vi "ControlShooter.vi"(1 "right down":T4, 2 "right up":T4, 3 "latch":T1={"DevStatus"={"status"=FALSE, "code"=0, "source"=""}, "Solenoid Module"=enum."Solenoid Module 1", "Forward Solenoid Channel"=enum."Invalid", "Reverse Solenoid Channel"=enum."Invalid"}, 4 "State":T8) -> ()   [LabVIEW 2013]
uses:
  typedefs/subStates.ctl
  <vilib>/Rock Robotics/WPI/Solenoid/WPI_SolenoidValue.ctl
  <vilib>/Rock Robotics/WPI/DigitalInput/WPI_DigitalInputDevRef.ctl
  <vilib>/Rock Robotics/SystemInterfaces/DIO/FPGA_DIOChannel.ctl
  <vilib>/Rock Robotics/SystemInterfaces/Typedef/FPGA_TypedefDigitalModule.ctl
  <vilib>/Rock Robotics/WPI/Solenoid/WPI_SolenoidDevRef.ctl
  <vilib>/Rock Robotics/SystemInterfaces/Typedef/FPGA_TypedefSolenoidModule.ctl
  <vilib>/Rock Robotics/WPI/Solenoid/WPI_SolenoidChannel.ctl
  typedefs/fg_typedef.ctl
  <vilib>/Rock Robotics/WPI/Solenoid/WPI_SolenoidGetEnum.vi
panel:
  out "To Shooter\nSolenoid Loop":T7=enum."Forward"
  # "unused"
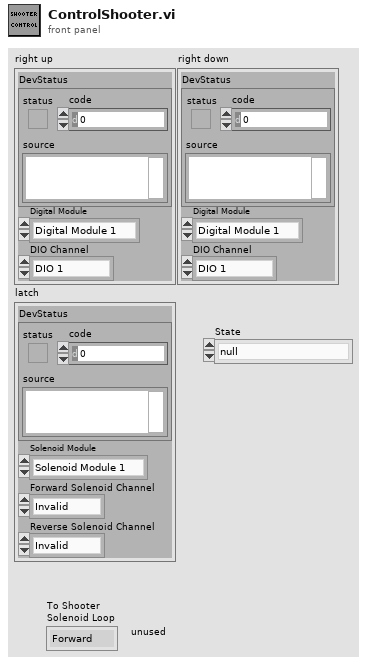
[diagram p1: front panel]
types:
  T1 = typedef "WPI_SolenoidDevRef.ctl" = cluster{"DevStatus":errorcluster, "Solenoid Module":T2, "Forward Solenoid Channel":T3, "Reverse Solenoid Channel":T3}
  T2 = typedef "FPGA_TypedefSolenoidModule.ctl" = enum16{"Solenoid Module 1", "Solenoid Module 2"}
  T3 = typedef "WPI_SolenoidChannel.ctl" = enum8{"Solenoid 1", "Solenoid 2", "Solenoid 3", "Solenoid 4", "Solenoid 5", "Solenoid 6", "Solenoid 7", "Solenoid 8", "Invalid"}
  T4 = typedef "WPI_DigitalInputDevRef.ctl" = cluster{"DevStatus":errorcluster, "DIO Channel":T5, "Digital Module":T6}
  T5 = typedef "FPGA_DIOChannel.ctl" = enum8{"DIO 1", "DIO 2", "DIO 3", "DIO 4", "DIO 5", "DIO 6", "DIO 7", "DIO 8", "DIO 9", "DIO 10", "DIO 11", "DIO 12", "DIO 13", "DIO 14", "Invalid"}
  T6 = typedef "FPGA_TypedefDigitalModule.ctl" = enum16{"Digital Module 1", "Digital Module 2"}
  T7 = typedef "WPI_SolenoidValue.ctl" = enum16{"Off", "On", "Forward", "Reverse"}
  T8 = typedef "subStates.ctl" = enum16{"null", "wait", "driver control", "auto", "manual override", "hold position", "rotate", "pickup", "pass", "load", "goto shoot", "shoot", "cancel", "end"}
  T9 = typedef "fg_typedef.ctl" = enum16{"Get", "Set"}
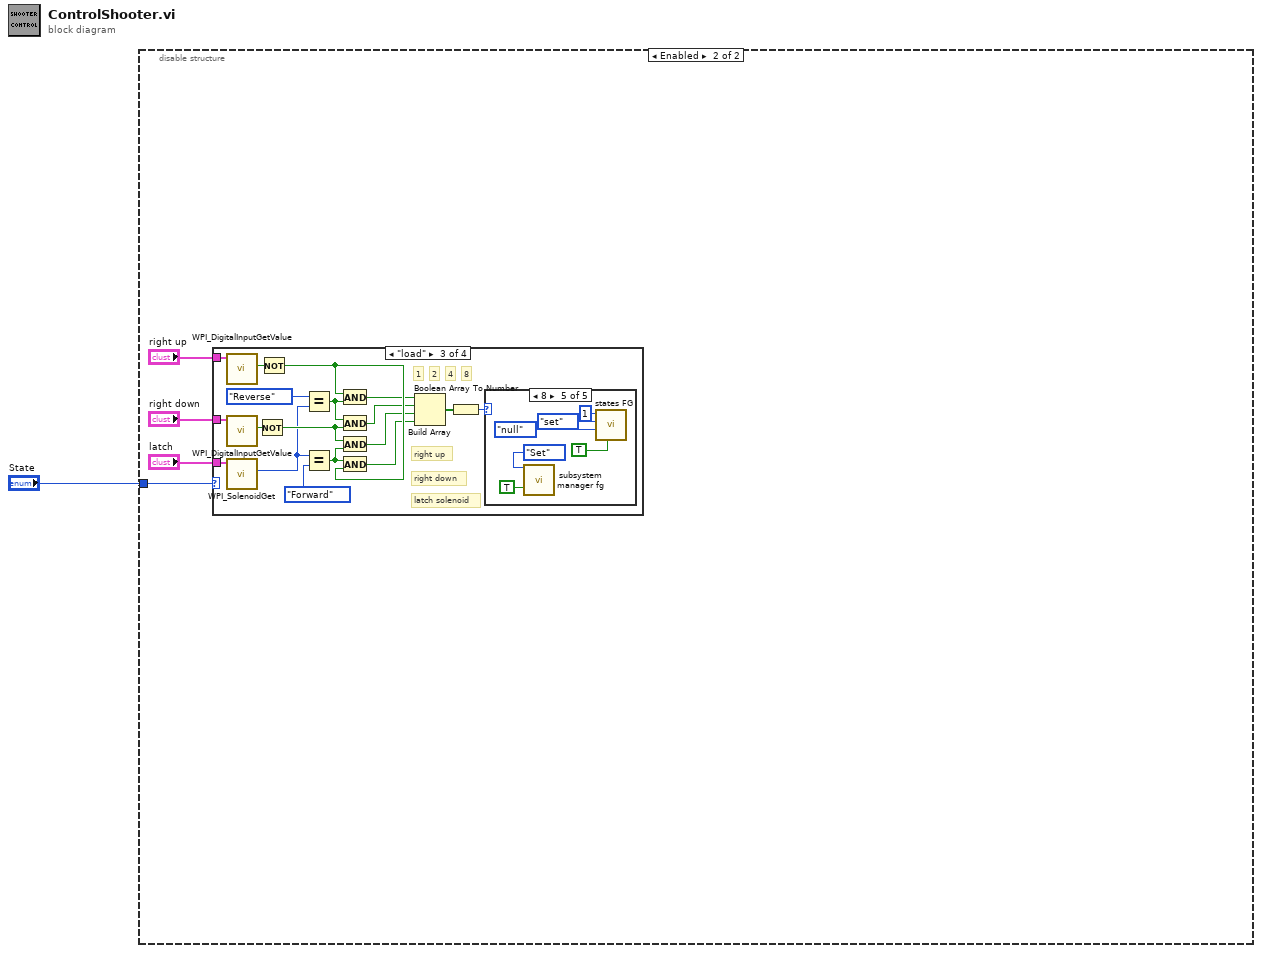
[diagram p0: block diagram]
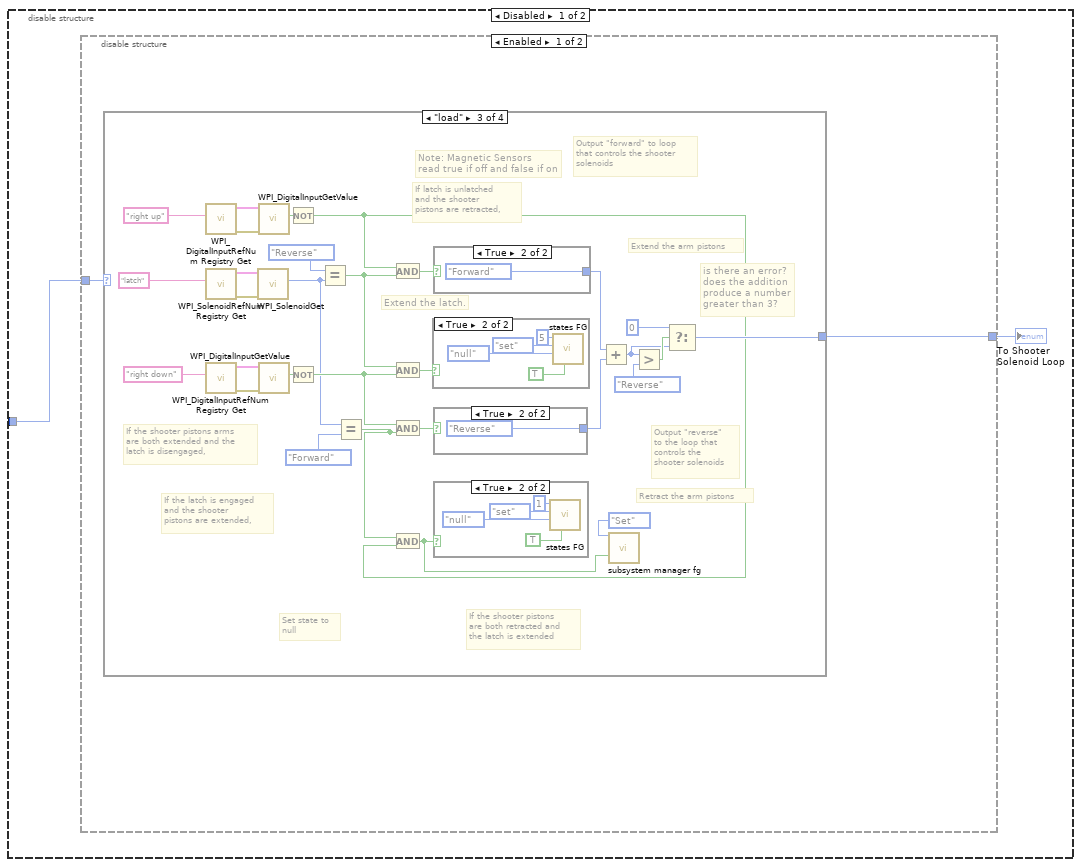
[diagram p2: hidden frame]
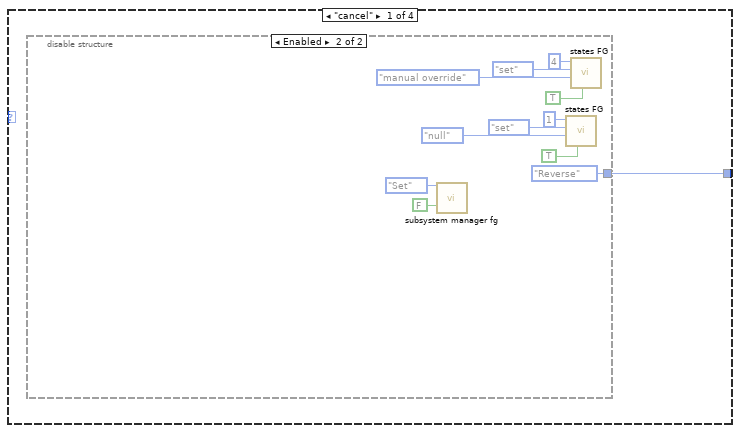
[diagram p3: hidden frame]
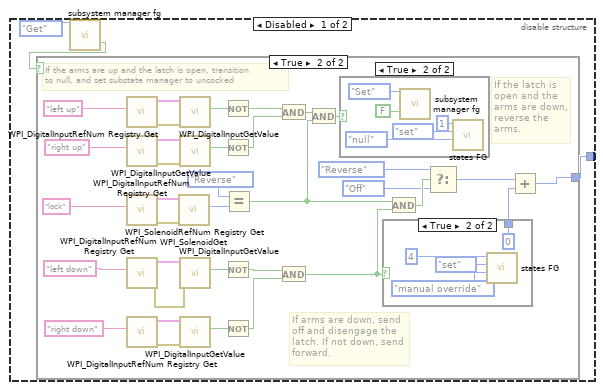
[diagram p4: hidden frame]
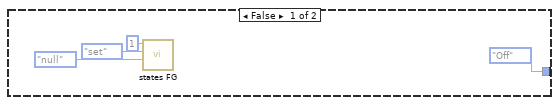
[diagram p5: hidden frame]
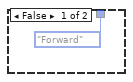
[diagram p7: hidden frame]
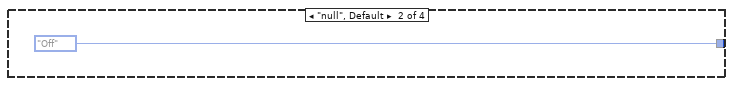
[diagram p8: hidden frame]
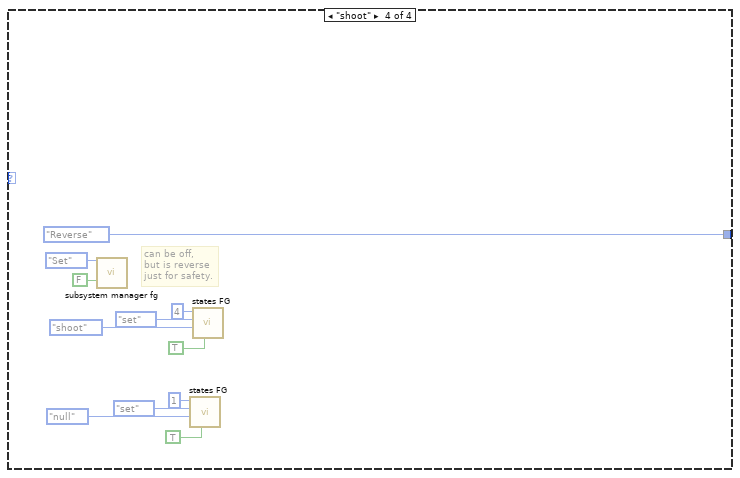
[diagram p13: hidden frame]
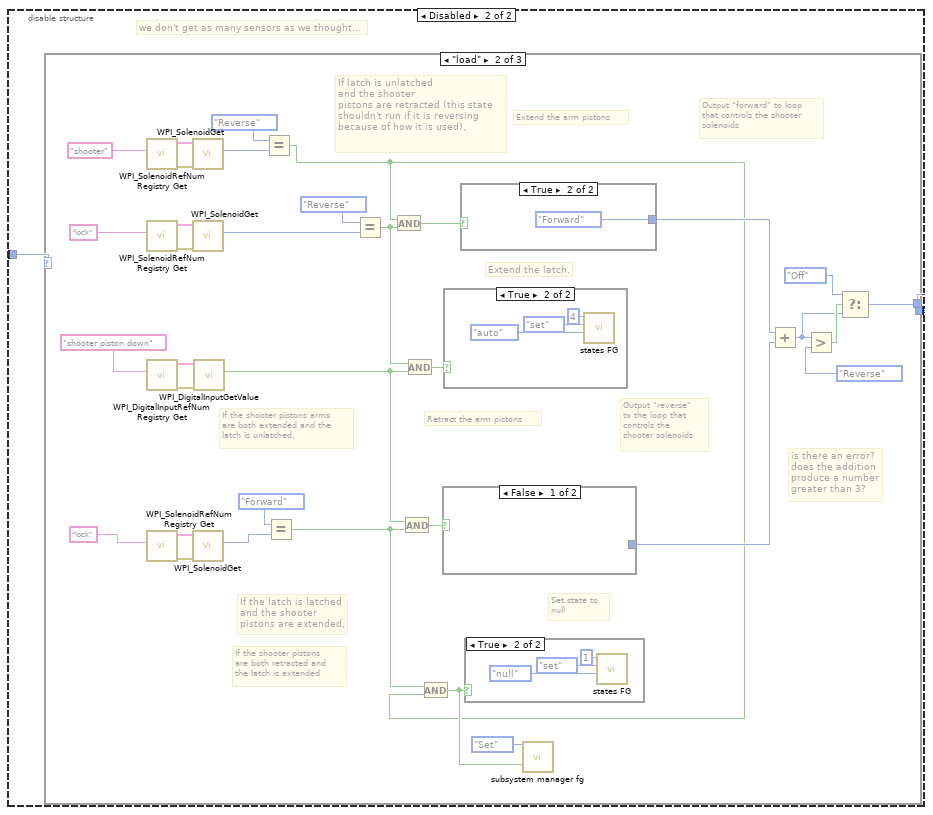
[diagram p14: hidden frame]
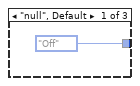
[diagram p15: hidden frame]
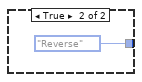
[diagram p17: hidden frame]
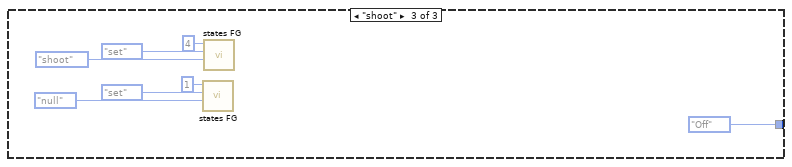
[diagram p20: hidden frame]
diagram:
  n1 = disable-structure shown="Enabled" {
    disable-tunnel: "State" -> [w3 w174]
    frame Disabled {
      n2 = disable-structure shown="Enabled" {
        disable-tunnel: w3 -> [w5 w123]
        disable-tunnel: [w4 w122] -> w2
        frame Enabled {
          n3 = case shown="\"load\"" w5 {
            tunnel: [w6 WPI_SolenoidValue."Off" ("To Shooter\nSolenoid Loop") w81 WPI_SolenoidValue."Reverse" ("To Shooter\nSolenoid Loop")] -> w4
            frame "cancel" {
              n4 = disable-structure shown="Enabled" {
                disable-tunnel: [w7 WPI_SolenoidValue."Reverse" ("To Shooter\nSolenoid Loop")] -> w6
                frame Disabled {
                  n5 = call "subsystem manager fg.vi"("Menu"=fg_typedef."Get") -> ("Shooter Cocked"=w8:bool)  [unwired: 14 in, 4 out]
                  n6 = case shown="True" w8 {
                    tunnel: [WPI_SolenoidValue."Off" ("To Shooter\nSolenoid Loop") w17] -> w7
                    frame False {
                      n7 = call "states FG.vi"("subState in"=subStates."null", "menu (get)"=enum16{"set", "get"}."set", "Loop ID"=1) -> ()  [unwired: 5 in, 4 out]
                    }
                    frame True {
                      # "If the arms are up and the latch is open, transition\nto null, and set substate manager to uncocked"
                      # "If the latch is\nopen and the\narms are down,\nreverse the\narms."
                      # "If arms are down, send\noff and disengage the\nlatch. If not down, send\nforward."
                      n8 = call <vilib>:"WPI_DigitalInputRefNum Registry Get.vi"("refnum name"="left up") -> ("error out"=w35:errorcluster, "DigitalInputDevRef"=w34:T4)  [unwired: 9 in]
                      n9 = call <vilib>:"WPI_DigitalInputRefNum Registry Get.vi"("refnum name"="right up") -> ("error out"=w32:errorcluster, "DigitalInputDevRef"=w31:T4)  [unwired: 9 in]
                      n10 = call <vilib>:"WPI_SolenoidRefNum Registry Get.vi"("refnum name"="lock") -> ("error out"=w28:errorcluster, "SolenoidDevRef"=w29:T1)  [unwired: 9 in]
                      n11 = call <vilib>:"WPI_DigitalInputRefNum Registry Get.vi"("refnum name"="left down") -> ("error out"=w38:errorcluster, "DigitalInputDevRef"=w37:T4)  [unwired: 9 in]
                      n12 = call <vilib>:"WPI_DigitalInputRefNum Registry Get.vi"("refnum name"="right down") -> ("error out"=w41:errorcluster, "DigitalInputDevRef"=w40:T4)  [unwired: 9 in]
                      n13 = call-poly <vilib>:"WPI_SolenoidGet.vi"("error in (no error)"=w28, "SolenoidDevRef"=w29) -> ("Value"=w47:T7)  [unwired: 7 in, 2 out]
                      n14 = call <vilib>:"WPI_DigitalInputGetValue.vi"("error in (no error)"=w35, "DigitalInputDevRef"=w34) -> ("Value"=w46:bool)  [unwired: 7 in, 2 out]
                      n15 = call <vilib>:"WPI_DigitalInputGetValue.vi"("error in (no error)"=w32, "DigitalInputDevRef"=w31) -> ("Value"=w45:bool)  [unwired: 7 in, 2 out]
                      n16 = call <vilib>:"WPI_DigitalInputGetValue.vi"("error in (no error)"=w38, "DigitalInputDevRef"=w37) -> ("Value"=w44:bool)  [unwired: 7 in, 2 out]
                      n17 = call <vilib>:"WPI_DigitalInputGetValue.vi"("error in (no error)"=w41, "DigitalInputDevRef"=w40) -> ("Value"=w43:bool)  [unwired: 7 in, 2 out]
                      n18 = Not(x=w46) -> (.not. x?=w26:bool)
                      n19 = Not(x=w45) -> (.not. x?=w27:bool)
                      n20 = Not(x=w44) -> (.not. x?=w24:bool)
                      n21 = Not(x=w43) -> (.not. x?=w25:bool)
                      n22 = Equal?(x=WPI_SolenoidValue."Reverse", y=w47) -> (x = y?=w15:bool)
                      n23 = And(x=w26, y=w27) -> (x .and. y?=w16:bool)
                      n24 = And(x=w24, y=w25) -> (x .and. y?=w23:bool)
                      n25 = And(x=w16, y=w15) -> (x .and. y?=w14:bool)
                      n26 = case shown="True" w14 {
                        frame False {
                        }
                        frame True {
                          n27 = call "subsystem manager fg.vi"("Menu"=fg_typedef."Set", "Shooter Cocked"=FALSE) -> ()  [unwired: 13 in, 5 out]
                          n28 = call "states FG.vi"("subState in"=subStates."null", "menu (get)"=enum16{"set", "get"}."set", "Loop ID"=1) -> ()  [unwired: 5 in, 4 out]
                        }
                      }
                      n29 = case shown="True" w23 {
                        tunnel: [WPI_SolenoidValue."Forward" ("To Shooter\nSolenoid Loop") 0] -> w22
                        frame False {
                        }
                        frame True {
                          n30 = call "states FG.vi"("subState in"=subStates."manual override", "menu (get)"=enum16{"set", "get"}."set", "Loop ID"=4) -> ()  [unwired: 5 in, 4 out]
                        }
                      }
                      n31 = And(x=w15, y=w23) -> (x .and. y?=w21:bool)
                      n32 = Select(t=WPI_SolenoidValue."Reverse" ("To Shooter\nSolenoid Loop"), s=w21, f=WPI_SolenoidValue."Off") -> (s? t:f=w19:T7)
                      n33 = Add(x=w19, y=w22) -> (x+y=w17:i32)
                    }
                  }
                }
                frame Enabled {
                  n34 = call "subsystem manager fg.vi"("Menu"=fg_typedef."Set", "Shooter Cocked"=FALSE) -> ()  [unwired: 13 in, 5 out]
                  n35 = call "states FG.vi"("exit in"=TRUE, "subState in"=subStates."null", "menu (get)"=enum16{"set", "get"}."set", "Loop ID"=1) -> ()  [unwired: 4 in, 4 out]
                  n36 = call "states FG.vi"("exit in"=TRUE, "subState in"=subStates."manual override", "menu (get)"=enum16{"set", "get"}."set", "Loop ID"=4) -> ()  [unwired: 4 in, 4 out]
                }
              }
            }
            frame "null", Default {
            }
            frame "load" {
              # "Note: Magnetic Sensors\nread true if off and false if on"
              # "is there an error?\ndoes the addition\nproduce a number \ngreater than 3?"
              # "Output \"reverse\"\nto the loop that\ncontrols the\nshooter solenoids"
              # "Output \"forward\" to loop\nthat controls the shooter\nsolenoids"
              # "Set state to\nnull"
              # "If the shooter pistons\nare both retracted and\nthe latch is extended"
              # "If the latch is engaged\nand the shooter\npistons are extended,"
              # "Retract the arm pistons"
              # "If latch is unlatched\nand the shooter\npistons are retracted,"
              # "Extend the latch."
              # "If the shooter pistons arms\nare both extended and the\nlatch is disengaged,"
              # "Extend the arm pistons"
              n37 = call <vilib>:"WPI_DigitalInputRefNum Registry Get.vi"("refnum name"="right up") -> ("error out"=w95:errorcluster, "DigitalInputDevRef"=w96:T4)  [unwired: 9 in]
              n38 = call <vilib>:"WPI_SolenoidRefNum Registry Get.vi"("refnum name"="latch") -> ("error out"=w100:errorcluster, "SolenoidDevRef"=w99:T1)  [unwired: 9 in]
              n39 = call <vilib>:"WPI_DigitalInputRefNum Registry Get.vi"("refnum name"="right down") -> ("error out"=w90:errorcluster, "DigitalInputDevRef"=w91:T4)  [unwired: 9 in]
              n40 = call-poly <vilib>:"WPI_SolenoidGet.vi"("error in (no error)"=w100, "SolenoidDevRef"=w99) -> ("Value"=w71:T7)  [unwired: 7 in, 2 out]
              n41 = call <vilib>:"WPI_DigitalInputGetValue.vi"("error in (no error)"=w95, "DigitalInputDevRef"=w96) -> ("Value"=w75:bool)  [unwired: 7 in, 2 out]
              n42 = call <vilib>:"WPI_DigitalInputGetValue.vi"("error in (no error)"=w90, "DigitalInputDevRef"=w91) -> ("Value"=w76:bool)  [unwired: 7 in, 2 out]
              n43 = Not(x=w75) -> (.not. x?=w74:bool)
              n44 = Not(x=w76) -> (.not. x?=w73:bool)
              n45 = Equal?(x=WPI_SolenoidValue."Reverse", y=w71) -> (x = y?=w87:bool)
              n46 = Equal?(x=w71, y=WPI_SolenoidValue."Forward" ("x")) -> (x = y?=w77:bool)
              n47 = And(x=w74, y=w87) -> (x .and. y?=w93:bool)
              n48 = And(x=w87, y=w73) -> (x .and. y?=w92:bool)
              n49 = And(x=w73, y=w77) -> (x .and. y?=w88:bool)
              n50 = And(x=w77, y=w74) -> (x .and. y?=w78:bool)
              n51 = case shown="True" w92 {
                frame False {
                }
                frame True {
                  n52 = call "states FG.vi"("exit in"=TRUE, "subState in"=subStates."null", "menu (get)"=enum16{"set", "get"}."set", "Loop ID"=5) -> ()  [unwired: 4 in, 4 out]
                }
              }
              n53 = case shown="True" w93 {
                tunnel: [_ WPI_SolenoidValue."Forward" ("Value")] -> w86
                frame False {
                }
                frame True {
                }
              }
              n54 = case shown="True" w88 {
                tunnel: [_ WPI_SolenoidValue."Reverse" ("Value")] -> w80
                frame False {
                }
                frame True {
                }
              }
              n55 = case shown="True" w78 {
                frame False {
                }
                frame True {
                  n56 = call "states FG.vi"("exit in"=TRUE, "subState in"=subStates."null", "menu (get)"=enum16{"set", "get"}."set", "Loop ID"=1) -> ()  [unwired: 4 in, 4 out]
                }
              }
              n57 = Add(x=w86, y=w80) -> (x+y=w83:u16)
              n58 = call "subsystem manager fg.vi"("Menu"=fg_typedef."Set", "Shooter Cocked"=w78) -> ()  [unwired: 13 in, 5 out]
              n59 = Greater?(x=w83, y=WPI_SolenoidValue."Reverse" ("Value")) -> (0:w84:bool)
              n60 = Select(t=0, s=w84, f=w83) -> (s? t:f=w81:i32)
            }
            frame "shoot" {
              # "can be off,\nbut is reverse\njust for safety."
              n61 = call "subsystem manager fg.vi"("Menu"=fg_typedef."Set", "Shooter Cocked"=FALSE) -> ()  [unwired: 13 in, 5 out]
              n62 = call "states FG.vi"("exit in"=TRUE, "subState in"=subStates."null", "menu (get)"=enum16{"set", "get"}."set", "Loop ID"=1) -> ()  [unwired: 4 in, 4 out]
              n63 = call "states FG.vi"("exit in"=TRUE, "subState in"=subStates."shoot", "menu (get)"=enum16{"set", "get"}."set", "Loop ID"=4) -> ()  [unwired: 4 in, 4 out]
            }
          }
        }
        frame Disabled {
          # "we don't get as many sensors as we thought..."
          n64 = case shown="\"load\"" w123 {
            tunnel: [WPI_SolenoidValue."Off" ("To Shooter\nSolenoid Loop") w136 WPI_SolenoidValue."Off" ("To Shooter\nSolenoid Loop")] -> w122
            frame "null", Default {
            }
            frame "load" {
              # "is there an error?\ndoes the addition\nproduce a number \ngreater than 3?"
              # "Output \"reverse\"\nto the loop that\ncontrols the\nshooter solenoids"
              # "Output \"forward\" to loop\nthat controls the shooter\nsolenoids"
              # "Set state to\nnull"
              # "If the shooter pistons\nare both retracted and\nthe latch is extended"
              # "If the latch is latched\nand the shooter\npistons are extended,"
              # "Retract the arm pistons"
              # "If latch is unlatched\nand the shooter\npistons are retracted (this state shouldn't run if it is reversing because of how it is used),"
              # "Extend the latch."
              # "If the shooter pistons arms\nare both extended and the\nlatch is unlatched,"
              # "Extend the arm pistons"
              n65 = call <vilib>:"WPI_SolenoidRefNum Registry Get.vi"("refnum name"="shooter") -> ("error out"=w128:errorcluster, "SolenoidDevRef"=w129:T1)  [unwired: 9 in]
              n66 = call <vilib>:"WPI_SolenoidRefNum Registry Get.vi"("refnum name"="lock") -> ("error out"=w158:errorcluster, "SolenoidDevRef"=w157:T1)  [unwired: 9 in]
              n67 = call <vilib>:"WPI_DigitalInputRefNum Registry Get.vi"("refnum name"="shooter piston down") -> ("error out"=w150:errorcluster, "DigitalInputDevRef"=w151:T4)  [unwired: 9 in]
              n68 = call <vilib>:"WPI_SolenoidRefNum Registry Get.vi"("refnum name"="lock") -> ("error out"=w148:errorcluster, "SolenoidDevRef"=w147:T1)  [unwired: 9 in]
              n69 = call-poly <vilib>:"WPI_SolenoidGet.vi"("error in (no error)"=w128, "SolenoidDevRef"=w129) -> ("Value"=w130:T7)  [unwired: 7 in, 2 out]
              n70 = call-poly <vilib>:"WPI_SolenoidGet.vi"("error in (no error)"=w158, "SolenoidDevRef"=w157) -> ("Value"=w155:T7)  [unwired: 7 in, 2 out]
              n71 = call-poly <vilib>:"WPI_SolenoidGet.vi"("error in (no error)"=w148, "SolenoidDevRef"=w147) -> ("Value"=w145:T7)  [unwired: 7 in, 2 out]
              n72 = call <vilib>:"WPI_DigitalInputGetValue.vi"("error in (no error)"=w150, "DigitalInputDevRef"=w151) -> ("Value"=w132:bool)  [unwired: 7 in, 2 out]
              n73 = Equal?(x=WPI_SolenoidValue."Reverse", y=w130) -> (x = y?=w126:bool)
              n74 = Equal?(x=WPI_SolenoidValue."Forward", y=w145) -> (x = y?=w141:bool)
              n75 = Equal?(x=WPI_SolenoidValue."Reverse", y=w155) -> (x = y?=w142:bool)
              n76 = And(x=w126, y=w142) -> (x .and. y?=w153:bool)
              n77 = And(x=w132, y=w141) -> (x .and. y?=w143:bool)
              n78 = And(x=w142, y=w132) -> (x .and. y?=w152:bool)
              n79 = And(x=w141, y=w126) -> (x .and. y?=w133:bool)
              n80 = case shown="False" w143 {
                tunnel: [_ WPI_SolenoidValue."Reverse" ("Value")] -> w135
                frame False {
                }
                frame True {
                }
              }
              n81 = case shown="True" w152 {
                frame False {
                }
                frame True {
                  n82 = call "states FG.vi"("subState in"=subStates."auto", "menu (get)"=enum16{"set", "get"}."set", "Loop ID"=4) -> ()  [unwired: 5 in, 4 out]
                }
              }
              n83 = case shown="True" w153 {
                tunnel: [_ WPI_SolenoidValue."Forward" ("Value")] -> w140
                frame False {
                }
                frame True {
                }
              }
              n84 = case shown="True" w133 {
                frame False {
                }
                frame True {
                  n85 = call "states FG.vi"("subState in"=subStates."null", "menu (get)"=enum16{"set", "get"}."set", "Loop ID"=1) -> ()  [unwired: 5 in, 4 out]
                }
              }
              n86 = call "subsystem manager fg.vi"("Menu"=fg_typedef."Set", "Shooter Cocked"=w133) -> ()  [unwired: 13 in, 5 out]
              n87 = Add(x=w140, y=w135) -> (x+y=w137:u16)
              n88 = Greater?(x=w137, y=WPI_SolenoidValue."Reverse" ("Value")) -> (0:w138:bool)
              n89 = Select(t=WPI_SolenoidValue."Off" ("Value"), s=w138, f=w137) -> (s? t:f=w136:u16)
            }
            frame "shoot" {
              n90 = call "states FG.vi"("subState in"=subStates."null", "menu (get)"=enum16{"set", "get"}."set", "Loop ID"=1) -> ()  [unwired: 5 in, 4 out]
              n91 = call "states FG.vi"("subState in"=subStates."shoot", "menu (get)"=enum16{"set", "get"}."set", "Loop ID"=4) -> ()  [unwired: 5 in, 4 out]
            }
          }
        }
      }
      "To Shooter\nSolenoid Loop" <- w2
    }
    frame Enabled {
      n92 = case shown="\"load\"" w174 {
        tunnel: "right up" -> [_ _ w192 _]
        tunnel: "right down" -> [_ _ w191 _]
        tunnel: "latch" -> [_ _ w190 _]
        frame "cancel" {
          # "retract shooter"
          # "unsafely open latch"
          n93 = call "subsystem manager fg.vi"("Menu"=fg_typedef."Set", "Shooter Cocked"=FALSE) -> ()  [unwired: 13 in, 5 out]
          n94 = call "states FG.vi"("exit in"=TRUE, "menu (get)"=enum16{"set", "get"}."set", "Loop ID"=5) -> ()  [unwired: 5 in, 4 out]
          n95 = call "states FG.vi"("exit in"=TRUE, "subState in"=subStates."null", "menu (get)"=enum16{"set", "get"}."set", "Loop ID"=1) -> ()  [unwired: 4 in, 4 out]
          n96 = call "states FG.vi"("exit in"=TRUE, "menu (get)"=enum16{"set", "get"}."set", "Loop ID"=5) -> ()  [unwired: 5 in, 4 out]
        }
        frame "null", Default {
        }
        frame "load" {
          # "latch solenoid"
          # "right down"
          # "right up"
          # "8"
          # "4"
          # "2"
          # "1"
          n97 = call <vilib>:"WPI_DigitalInputGetValue.vi"("DigitalInputDevRef"=w192) -> ("Value"=w203:bool)  [unwired: 8 in, 2 out]
          n98 = call <vilib>:"WPI_DigitalInputGetValue.vi"("DigitalInputDevRef"=w191) -> ("Value"=w204:bool)  [unwired: 8 in, 2 out]
          n99 = call-poly <vilib>:"WPI_SolenoidGet.vi"("SolenoidDevRef"=w190) -> ("Value"=w193:T7)  [unwired: 8 in, 2 out]
          n100 = Not(x=w204) -> (.not. x?=w201:bool)
          n101 = Not(x=w203) -> (.not. x?=w202:bool)
          n102 = Equal?(x=WPI_SolenoidValue."Reverse", y=w193) -> (x = y?=w206:bool)
          n103 = Equal?(x=w193, y=WPI_SolenoidValue."Forward" ("x")) -> (x = y?=w205:bool)
          n104 = And(x=w202, y=w206) -> (x .and. y?=w200:bool)
          n105 = And(x=w206, y=w201) -> (x .and. y?=w199:bool)
          n106 = And(x=w201, y=w205) -> (x .and. y?=w198:bool)
          n107 = And(x=w205, y=w202) -> (x .and. y?=w197:bool)
          n108 = Build Array(w200, w199, w198, w197) -> (w196:bool[])
          n109 = Boolean Array To Number(Boolean array=w196) -> (number=w195:u32)
          n110 = case shown="8" w195 {
            frame 0, Default {
            }
            frame 1 {
              # "extend shooter"
              n111 = call "states FG.vi"("exit in"=FALSE, "menu (get)"=enum16{"set", "get"}."set", "Loop ID"=5) -> ()  [unwired: 5 in, 4 out]
            }
            frame 2 {
              # "close latch"
              n112 = call "states FG.vi"("exit in"=FALSE, "menu (get)"=enum16{"set", "get"}."set", "Loop ID"=5) -> ()  [unwired: 5 in, 4 out]
            }
            frame 4 {
              # "retract shooter"
              n113 = call "states FG.vi"("exit in"=FALSE, "menu (get)"=enum16{"set", "get"}."set", "Loop ID"=5) -> ()  [unwired: 5 in, 4 out]
            }
            frame 8 {
              n114 = call "subsystem manager fg.vi"("Menu"=fg_typedef."Set", "Shooter Cocked"=TRUE) -> ()  [unwired: 13 in, 5 out]
              n115 = call "states FG.vi"("exit in"=TRUE, "subState in"=subStates."null", "menu (get)"=enum16{"set", "get"}."set", "Loop ID"=1) -> ()  [unwired: 4 in, 4 out]
            }
          }
        }
        frame "shoot" {
          # "retract shooter"
          # "open latch"
          # "can be off,\nbut is reverse\njust for safety."
          n116 = call "subsystem manager fg.vi"("Menu"=fg_typedef."Set", "Shooter Cocked"=FALSE) -> ()  [unwired: 13 in, 5 out]
          n117 = call "states FG.vi"("exit in"=TRUE, "menu (get)"=enum16{"set", "get"}."set", "Loop ID"=5) -> ()  [unwired: 5 in, 4 out]
          n118 = call "states FG.vi"("exit in"=TRUE, "subState in"=subStates."null", "menu (get)"=enum16{"set", "get"}."set", "Loop ID"=1) -> ()  [unwired: 4 in, 4 out]
          n119 = call "states FG.vi"("exit in"=TRUE, "menu (get)"=enum16{"set", "get"}."set", "Loop ID"=5) -> ()  [unwired: 5 in, 4 out]
        }
      }
    }
  }
